vi "Online_Target.vi"   [LabVIEW 2021]
uses:
  Model_Updating_Classes/DROPBEAR_Model_Updating/DROPBEAR_Model_Updating.lvclass
  Model_Updating_Classes/MOCKBEAR/MOCKBEAR.lvclass
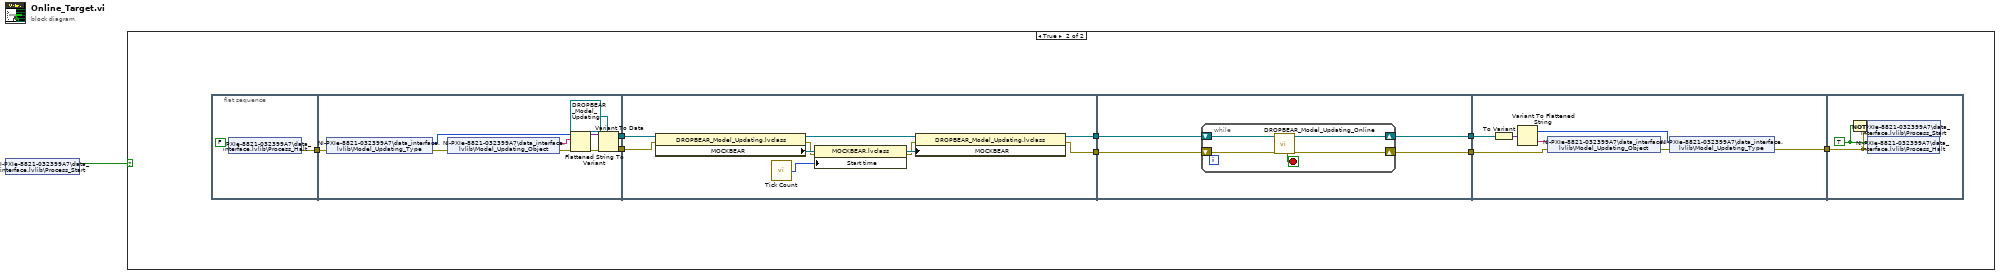
[diagram p0: block diagram]
diagram:
  n1 = shared-variable "NI-PXIe-8821-032399A7\\data_interface.lvlib\\Process_Start"() -> (w1:bool)  [unwired: 1 in, 1 out]
  n2 = case shown="True" w1 {
    frame False {
    }
    frame True {
      n3 = flat-sequence {
        tunnel: [w10] -> w9
        tunnel: [w14] -> w8
        tunnel: [w15] -> w7
        tunnel: w9 -> [w12]
        tunnel: w8 -> [w22]
        tunnel: [w25] -> w6
        tunnel: w7 -> [w26]
        tunnel: [w24] -> w5
        tunnel: w6 -> [w35]
        tunnel: [w34] -> w4
        tunnel: w5 -> [w33]
        tunnel: [w32] -> w3
        tunnel: w4 -> [w47]
        tunnel: w3 -> [w42]
        tunnel: [w41] -> w2
        tunnel: w2 -> [w48]
        frame #0 {
          n4 = shared-variable "NI-PXIe-8821-032399A7\\data_interface.lvlib\\Process_Halt"(FALSE ("Process_Halt")) -> (error out=w10:errorcluster)  [unwired: 1 in]
        }
        frame #1 {
          n5 = shared-variable "NI-PXIe-8821-032399A7\\data_interface.lvlib\\Model_Updating_Type"(error in=w12) -> (w19:i16[], error out=w16:errorcluster)
          n6 = shared-variable "NI-PXIe-8821-032399A7\\data_interface.lvlib\\Model_Updating_Object"(error in=w16) -> (w18:string, error out=w17:errorcluster)
          n7 = Flattened String To Variant(4:w17, 6:w18, 7:w19) -> (0:w21:errorcluster, 3:w20:variant)
          n8 = Variant To Data(error in=w21, type=refnum<class "DROPBEAR_Model_Updating.lvclass"> refnum ("DROPBEAR_Model_Updating.lvclass"), Variant=w20) -> (data=w14:refnum<class "DROPBEAR_Model_Updating.lvclass">, error out=w15:errorcluster)
        }
        frame #2 {
          n9 = property class="DROPBEAR_Model_Updating.lvclass"(reference=w22, error in=w26) -> (reference out=w29:refnum<class "DROPBEAR_Model_Updating.lvclass">, error out=w23:errorcluster, "MOCKBEAR"=w31:refnum<class "MOCKBEAR.lvclass">)
          n10 = call "Tick Count"() -> ("Tick Count(uSec)"=w28:u32)
          n11 = property class="MOCKBEAR.lvclass"(reference=w31, error in=w23, "Start time"=w28) -> (reference out=w30:refnum<class "MOCKBEAR.lvclass">, error out=w27:errorcluster)
          n12 = property class="DROPBEAR_Model_Updating.lvclass"(reference=w29, error in=w27, "MOCKBEAR"=w30) -> (reference out=w25:refnum<class "DROPBEAR_Model_Updating.lvclass">, error out=w24:errorcluster)
        }
        frame #3 {
          n13 = while {
            shift-right: [w38] -> w34
            shift-left: w35 -> [w40]
            shift-right: [w37] -> w32
            shift-left: w33 -> [w39]
            stop <- w36 stop-if-true
            n14 = call-dynamic "DROPBEAR_Model_Updating_Online.vi"("error in (no error)"=w39, "DROPBEAR_Model_Updating in"=w40) -> ("error out"=w37:errorcluster, "DROPBEAR_Model_Updating out"=w38:refnum<class "DROPBEAR_Model_Updating.lvclass">, "looping"=w36:bool)  [unwired: 7 in]
          }
        }
        frame #4 {
          n15 = To Variant(anything=w47) -> (Variant=w43:variant)
          n16 = Variant To Flattened String(Variant=w43) -> (data string=w46:string, 1:w44:i16[])
          n17 = shared-variable "NI-PXIe-8821-032399A7\\data_interface.lvlib\\Model_Updating_Object"(w46, error in=w42) -> (error out=w45:errorcluster)
          n18 = shared-variable "NI-PXIe-8821-032399A7\\data_interface.lvlib\\Model_Updating_Type"(w44, error in=w45) -> (error out=w41:errorcluster)
        }
        frame #5 {
          w50 = TRUE ("Process_Halt")
          n19 = Not(x=w50) -> (.not. x?=w49:bool)
          n20 = shared-variable "NI-PXIe-8821-032399A7\\data_interface.lvlib\\Process_Start"(w49, error in=w48) -> ()  [unwired: 1 out]
          n21 = shared-variable "NI-PXIe-8821-032399A7\\data_interface.lvlib\\Process_Halt"(w50, error in=w48) -> ()  [unwired: 1 out]
        }
      }
    }
  }
